vi "Vision Processing.vi"(4 "error in (no error)":errorcluster, 7 "Image Size":T1=enum."320x240") -> ()   [LabVIEW 2015]
doc: "This VI runs in parallel to other tasks. It gets images from the camera, processes them for color or shape and use that information to affect robot behavior."
uses:
  <vilib>/Rock Robotics/WPI/Camera/WPI_CameraImageSize.ctl
  <vilib>/vision/Image Controls.llb/IMAQ Image.ctl
  Program Files (x86)/National Instruments/LabVIEW 2015/examples/FRC/roboRIO/Vision/2016 Vision Example/Vision Support Code/Camera Types.ctl
  <vilib>/Rock Robotics/WPI/Camera/WPI_CameraWhite Balance Values.ctl
  <vilib>/Rock Robotics/WPI/Camera/WPI_CameraFrameRate.ctl
  <vilib>/Rock Robotics/WPI/Camera/WPI_CameraExposure Values.ctl
  Robot Global Data.vi
  Team Code/Global_Var/Drive_Global.vi
  <vilib>/vision/NI_Vision_Development_Module.lvlib
panel:
  out "Waveform Chart":dbl(graph)
  out "Vision_angle":cluster{"1":dbl, "2":dbl, "3":dbl}
  in  "Snap_Shot":bool
  in  "error in (no error) 2":errorcluster
  in  "Image Size 2":T1
  out "ms to process":u32=51
  in  "LED Color":T2={"Hue"={238.51289036032986, 17.562943497940463}, "Sat"={66.78571428571429, 255.0}, "Val"={48.571428571428584, 255.0}} {"Hue" scale=0.0..255.0 scale format="%#_3g"}
  out "Qualified Particles":i32
  in  "Score Threshold":dbl=75.0
  in  "Aspect Fudge Factor":dbl=1.0
  in  "Min Score Threshold":i32=75
  in  "Camera Type":T3=enum."MS HD3000 square"
  in  "Emphasize Limit Tests":bool=TRUE
  out "Masked 2":T4(plugin-control)
  in  "Display Mask":bool=TRUE
  out "Original Image":T4(plugin-control)
  in  "Display Original":bool=TRUE
  out "Sorted Particle Scores":T5(array[cluster]) {"Moment Factor" format="%#_3g"; "Aspect Ratio" format="%#_3g"; "Area to CH" format="%#_3g"; "X" format="%#_3g"; "Y" format="%#_3g"}
  out "Highest Avg Score":dbl
  out "Detected Targets":T6(array[cluster]) {"Normalized Rect"."Numeric 5" format="%#_2g"; "Normalized Rect"."Numeric 3" format="%#_2g"; "Normalized Rect"."Numeric 2" format="%#_2g"; "Normalized Rect"."Numeric" format="%#_2g"}
  out "fps":dbl=19.607843137254903
  out "Image Out":T4
  # "Density Profile"
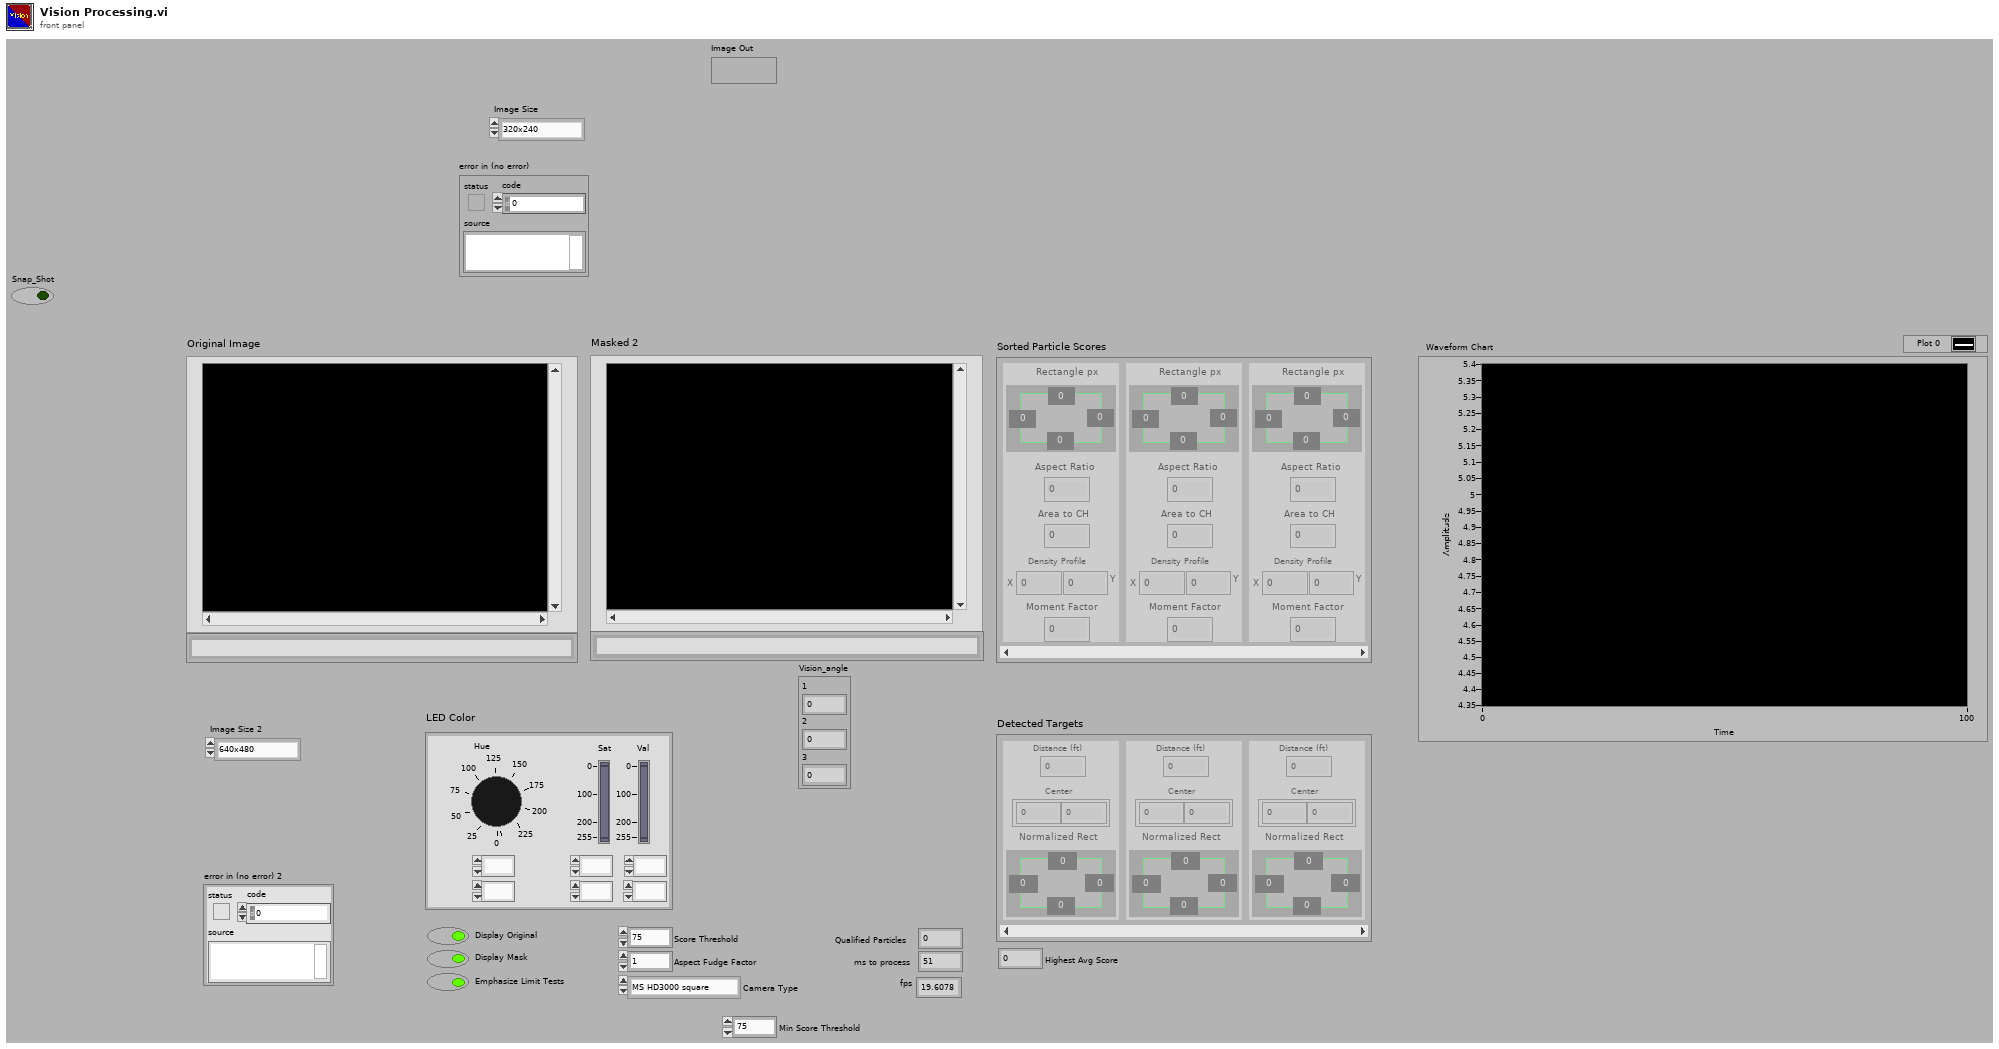
[diagram p1: front panel]
types:
  T1 = typedef "WPI_CameraImageSize.ctl" = enum16{"640x480", "320x240", "160x120", "Custom"}
  T2 = cluster{"Hue":cluster{dbl, dbl}, "Sat":cluster{dbl, dbl}, "Val":cluster{dbl, dbl}}
  T3 = typedef "Camera Types.ctl" = enum16{"206", "1011", "1013", "MS HD3000 square", "MS HD3000 640x480"}
  T4 = typedef "IMAQ Image.ctl" = refnum<image>
  T5 = cluster{"Rectangle px":cluster{"Numeric":dbl, "Numeric 2":dbl, "Numeric 3":dbl, "Numeric 5":dbl}, "Aspect Ratio":dbl, "Area to CH":dbl, "X":dbl, "Y":dbl, "Moment Factor":dbl}[]
  T6 = cluster{"Distance (ft)":dbl, "Center":cluster{dbl, dbl}, "Normalized Rect":cluster{"Numeric":dbl, "Numeric 2":dbl, "Numeric 3":dbl, "Numeric 5":dbl}}[]
  T7 = typedef "WPI_CameraExposure Values.ctl" = enum16{"Auto", "Flicker-free 50 Hz", "Flicker-free 60 Hz", "Hold current", "Custom"}
  T8 = typedef "WPI_CameraFrameRate.ctl" = u32
  T9 = typedef "WPI_CameraWhite Balance Values.ctl" = enum16{"Auto", "Fixed indoor", "Fixed outdoor 1", "Fixed outdoor 2", "Fixed fluorescent 1", "Fixed fluorescent 2", "Hold current", "Custom"}
  T10 = enum16{"Rising", "Falling", "Falling and Rising"}
  T11 = typedef "Particle Parameters" = i32
  T12 = typedef "Image Type" = u32
  T13 = typedef "WPI_CameraDevRef.ctl" = cluster{"Camera Address":string, "CameraStatus":errorcluster}
  T14 = cluster{"Bounding box":cluster{"left":dbl, "top":dbl, "right":dbl, "bottom":dbl}, "Aspect Ratio":dbl, "Area to CH":dbl, "X Mask":dbl, "Y Mask":dbl, "Moment":dbl}[]
  T15 = cluster{"Rectangle":cluster{"Numeric":dbl, "Numeric 2":dbl, "Numeric 3":dbl, "Numeric 5":dbl}, "L":dbl, "Area to CH":dbl, "X":dbl, "Y":dbl, "Moment Factor":dbl}[]
  T16 = cluster{"Distance (ft)":dbl, "Center":cluster{dbl, dbl}, "Normalized Rect":cluster{"Numeric":dbl, "Numeric 2":dbl, "Numeric 3":dbl, "Numeric 5":dbl}}
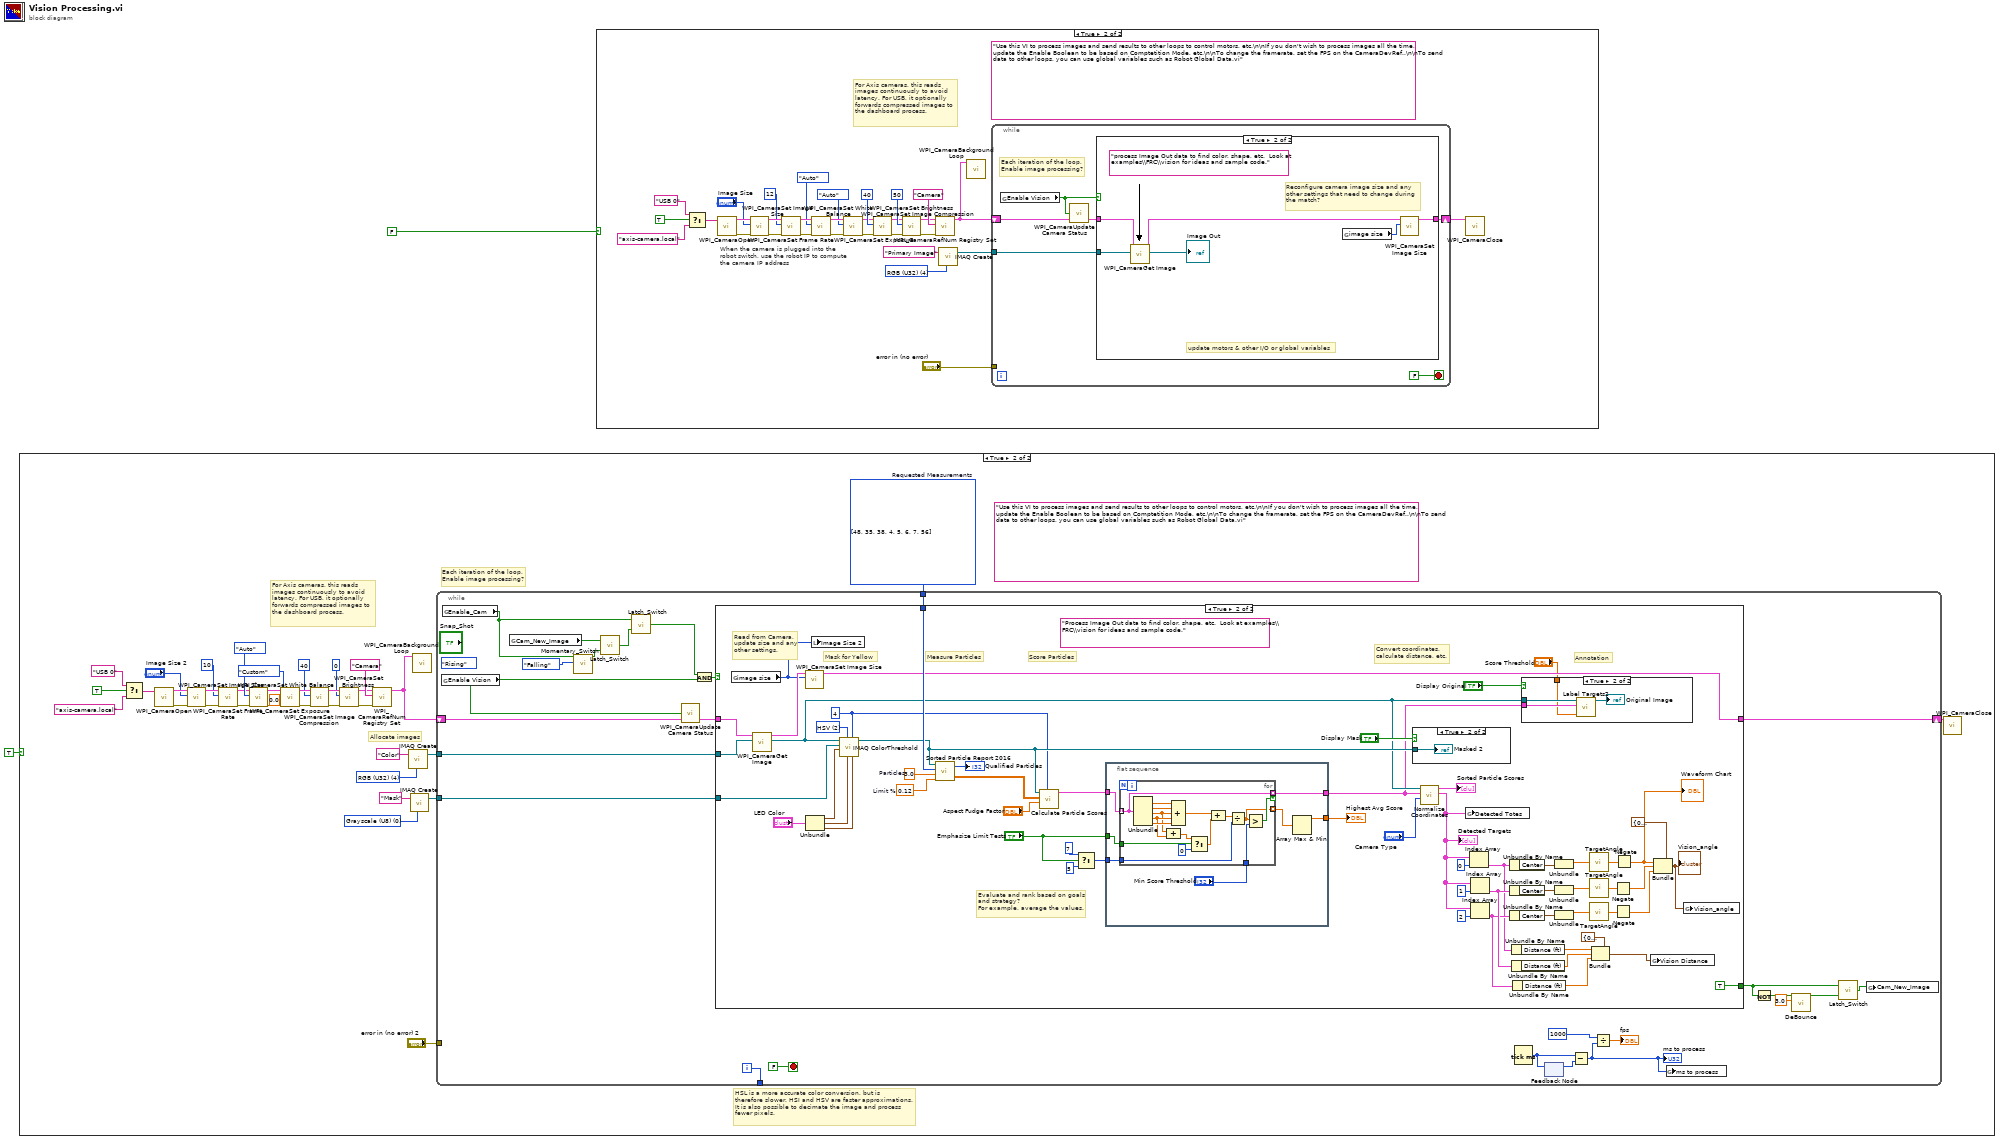
[diagram p0: block diagram]
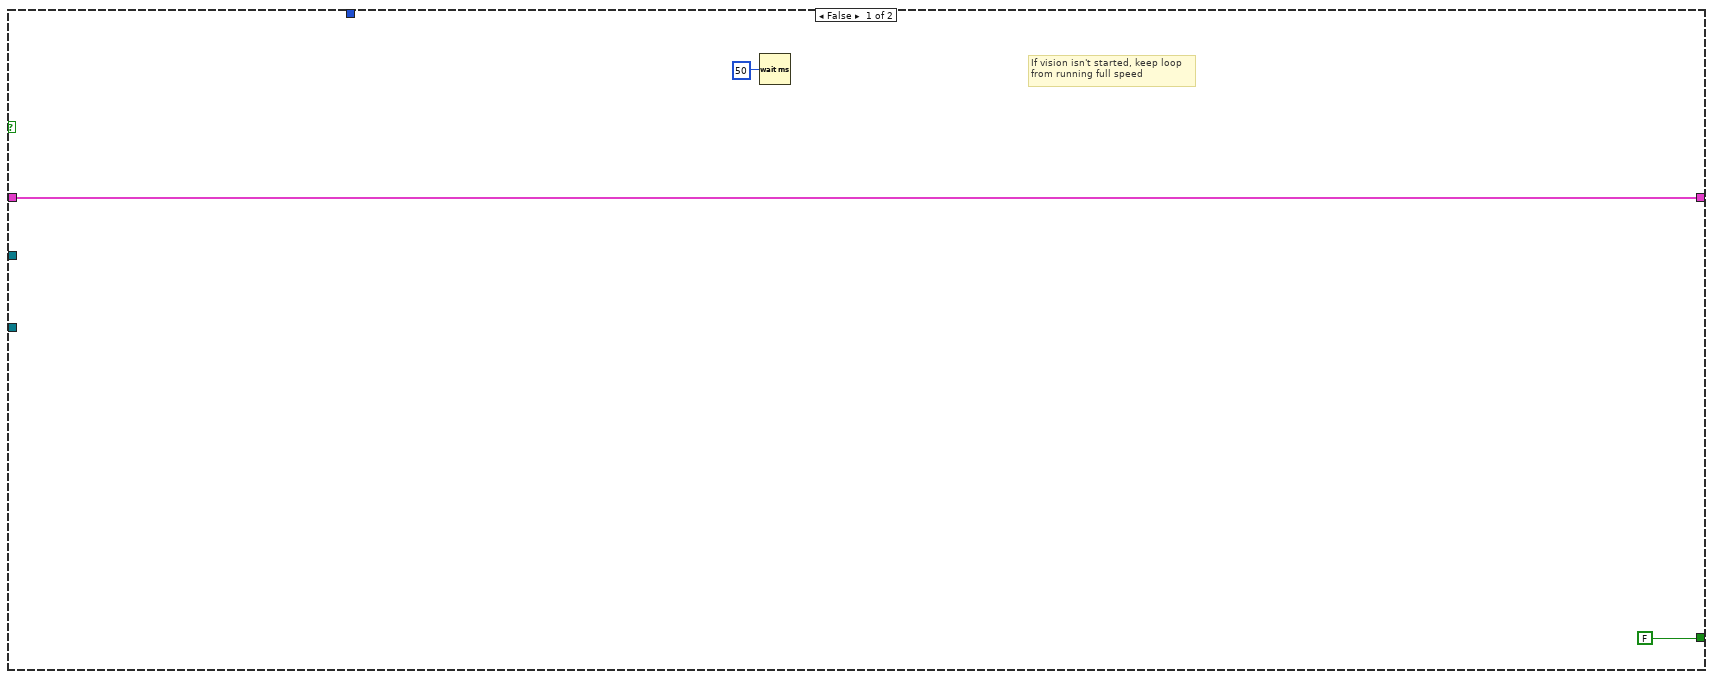
[diagram p3: hidden frame]
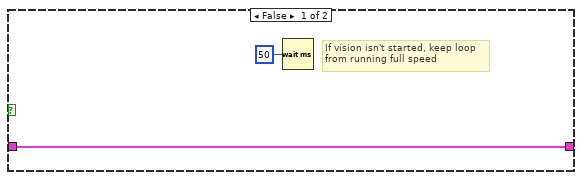
[diagram p7: hidden frame]
diagram:
  n1 = case shown="True" TRUE {
    frame False {
    }
    frame True {
      (unwired) "Use this VI to process images and send results to other loops to control motors, etc.\n\nIf you don't wish to process images all the time, update the Enable Boolean to be based on Comptetition Mode, etc.\n\nTo change the framerate, set the FPS on the CameraDevRef..\n\nTo send data to other loops, you can use global variables such as Robot Global Data.vi"
      w32 = T11[] [48, 35, 38, 4, 5, 6, 7, 56] items=["Center of Mass X", "Center of Mass Y", "First Pixel X", "First Pixel Y", "Bounding Rect Left", "Bounding Rect Top", "Bounding Rect Right", "Bounding Rect Bottom", "Max Feret Diameter Start X", "Max Feret Diameter Start Y", "Max Feret Diameter End X", "Max Feret Diameter End Y", "Max Horiz. Segment Length Left", "Max Horiz. Segment Length Right", "Max Horiz. Segment Length Row", "-", "Bounding Rect Width", "Bounding Rect Height", "Bounding Rect Diagonal", "Perimeter", "Convex Hull Perimeter", "Holes' Perimeter", "Max Feret Diameter", "Equivalent Ellipse Major Axis", "Equivalent Ellipse Minor Axis", "Equivalent Ellipse Minor Axis (Feret)", "Equivalent Rect Long Side", "Equivalent Rect Short Side", "Equivalent Rect Diagonal", "Equivalent Rect Short Side (Feret)", "Average Horiz. Segment Length", "Average Vert. Segment Length", "Hydraulic Radius", "Waddel Disk Diameter", "-", "Area", "Holes' Area", "Particle & Holes' Area", "Convex Hull Area", "Image Area", "-", "Number of Holes", "Number of Horiz. Segments", "Number of Vert. Segments", "-", "Orientation", "Max Feret Diameter Orientation", "-", "% Area/Image Area", "% Area/(Particle & Holes' Area)", "Ratio of Equivalent Ellipse Axes", "Ratio of Equivalent Rect Sides", "-", "Elongation Factor", "Compactness Factor", "Heywood Circularity Factor", "Type Factor", "-", "Sum X", "Sum Y", "Sum XX", "Sum XY", "Sum YY", "Sum XXX", "Sum XXY", "Sum XYY", "Sum YYY", "-", "Moment of Inertia XX", "Moment of Inertia XY", "Moment of Inertia YY", "Moment of Inertia XXX", "Moment of Inertia XXY", "Moment of Inertia XYY", "Moment of Inertia YYY", "Norm. Moment of Inertia XX", "Norm. Moment of Inertia XY", "Norm. Moment of Inertia YY", "Norm. Moment of Inertia XXX", "Norm. Moment of Inertia XXY", "Norm. Moment of Inertia XYY", "Norm. Moment of Inertia YYY", "Hu Moment 1", "Hu Moment 2", "Hu Moment 3", "Hu Moment 4", "Hu Moment 5", "Hu Moment 6", "Hu Moment 7"]  # Requested Measurements
      w35 = T12 0 items=["Grayscale (U8)", "Grayscale (I16)", "Grayscale (SGL)", "Complex (CSG)", "RGB (U32)", "HSL (U32)", "RGB (U64)", "Grayscale (U16)"] ("Image Type")
      w37 = T12 4 items=["Grayscale (U8)", "Grayscale (I16)", "Grayscale (SGL)", "Complex (CSG)", "RGB (U32)", "HSL (U32)", "RGB (U64)", "Grayscale (U16)"] ("Image Type")
      # "Each iteration of the loop,\nEnable image processing?"
      # "HSL is a more accurate color conversion, but is\ntherefore slower. HSI and HSV are faster approximations.\nIt is also possible to decimate the image and process\nfewer pixels."
      # "For Axis cameras, this reads\nimages continuously to avoid\nlatency. For USB, it optionally\nforwards compressed images to\nthe dashboard process."
      # "Allocate images"
      n2 = Select(t="USB 0" ("format string"), s=TRUE ("dot notation? (F)"), f="axis-camera.local" ("format string")) -> (s? t:f=w31:string)
      n3 = call <vilib>:"WPI_CameraOpen.vi"("Camera Address"=w31) -> ("error out"=w21:errorcluster, "CameraDevRef"=w20:T13)  [unwired: 1 in, 8 out]
      n4 = call <vilib>:"WPI_CameraSet Image Size.vi"("error in (no error)"=w21, "Image Size"="Image Size 2", "CameraDevRef"=w20) -> ("error out"=w22:errorcluster, "CameraDevRef Out"=w19:T13)  [unwired: 1 in, 6 out]
      n5 = call <vilib>:"WPI_CameraSet Frame Rate.vi"("error in (no error)"=w22, "Frame Rate (fps)"=T8 10, "CameraDevRef"=w19) -> ("error out"=w23:errorcluster, "CameraDevRef Out"=w17:T13)  [unwired: 7 out]
      n6 = call <vilib>:"WPI_CameraSet White Balance.vi"("error in (no error)"=w23, "White Balance"=WPI_CameraWhite_Balance_Values."Auto", "CameraDevRef"=w17) -> ("error out"=w24:errorcluster, "CameraDevRef Out"=w18:T13)  [unwired: 1 in, 6 out]
      n7 = call <vilib>:"WPI_CameraSet Exposure.vi"("error in (no error)"=w24, "Exposure (%)"=0.0, "Exposure"=WPI_CameraExposure_Values."Custom", "CameraDevRef"=w18) -> ("error out"=w25:errorcluster, "CameraDevRef Out"=w15:T13)  [unwired: 6 out]
      n8 = call <vilib>:"WPI_CameraSet Image Compression.vi"("error in (no error)"=w25, "Compression"=40, "CameraDevRef"=w15) -> ("error out"=w26:errorcluster, "CameraDevRef Out"=w16:T13)  [unwired: 7 out]
      n9 = call <vilib>:"WPI_CameraSet Brightness.vi"("error in (no error)"=w26, "Brightness"=0, "CameraDevRef"=w16) -> ("error out"=w27:errorcluster, "CameraDevRef Out"=w6:T13)  [unwired: 7 out]
      n10 = call <vilib>:"WPI_CameraRefNum Registry Set.vi"("error in (no error)"=w27, "refnum name"="Camera", "CameraDevRef"=w6) -> ("CameraDevRef"=w11:T13)  [unwired: 1 in, 7 out]
      n11 = call "IMAQ Create"("Image Name"="Color", "Image Type"=w37) -> ("New Image"=w36:T4)  [unwired: 2 in, 2 out]
      n12 = call "IMAQ Create"("Image Name"="Mask", "Image Type"=w35) -> ("New Image"=w33:T4)  [unwired: 2 in, 2 out]
      n13 = call <vilib>:"WPI_CameraBackground Loop.vi"("CameraDevRef"=w11) -> ()  [unwired: 11 in]
      n14 = while {
        tunnel: w36 -> [w59]
        tunnel: w33 -> [w63]
        tunnel: w32 -> [w62]
        tunnel: "error in (no error) 2" -> [_]
        tunnel: [w58] -> _
        shift-right: [w55] -> w7
        shift-left: w11 -> [w57]
        i -> [w58]
        stop <- FALSE stop-if-true
        (unwired) T10."Rising" ("Type")
        n15 = global read "Robot Global Data.vi" "Enable Vision"() -> (w51:bool)
        n16 = global read "Drive_Global.vi" "Enable_Cam"() -> (w47:bool)
        n17 = global read "Drive_Global.vi" "Cam_New_Image"() -> (w45:bool)
        n18 = call "Momentary_Switch.vi"("Type"=T10."Falling", "input_bol"=w47) -> ("out"=w50:bool)  [unwired: 9 in]
        n19 = call "Latch_Switch.vi"("Reset"=w50, "In"=w45) -> ("Out"=w48:bool)
        n20 = call "Latch_Switch.vi"("Reset"=w48, "In"=w47) -> ("Out"=w46:bool)
        n21 = call <vilib>:"WPI_CameraUpdate Camera Status.vi"("CameraDevRef In"=w57, "Enable Vision"=w51) -> ("CameraDevRef Out"=w56:T13)  [unwired: 3 in]
        n22 = And(x=w46, y=w51) -> (x .and. y?=w39:bool)
        n23 = case shown="True" w39 {
          tunnel: w63 -> [_ w126]
          tunnel: w62 -> [_ w121]
          tunnel: w56 -> [w66 w117]
          tunnel: w59 -> [_ w116]
          tunnel: [w66 w114] -> w55
          tunnel: [FALSE TRUE] -> w40
          frame False {
            # "If vision isn't started, keep loop\nfrom running full speed"
            n24 = Wait (ms)(milliseconds to wait=u32 50) -> ()  [unwired: 1 out]
          }
          frame True {
            w97 = 4 ("Replace Value")
            w111 = u16 2 items=["RGB", "HSL", "HSV", "HSI"] ("Color Mode")
            (unwired) "Process Image Out data to find color, shape, etc.  Look at examples\\FRC\\vision for ideas and sample code."
            w118 = 0.12  # Limit %
            w120 = 3.0  # Particles
            # "Evaluate and rank based on goals\nand strategy?\nFor example, average the values."
            # "Read from Camera,\nupdate size and any\nother settings."
            # "Measure Particles"
            # "Convert coordinates,\ncalculate distance, etc."
            # "Annotation"
            # "Score Particles"
            # "Mask for Yellow"
            n25 = global read "Robot Global Data.vi" "image size"() -> (w96:T1)
            n26 = call <vilib>:"WPI_CameraGet Image.vi"("Image"=w116, "CameraDevRef"=w117) -> ("Image Out"=w100:T4, "CameraDevRef Out"=w115:T13)  [unwired: 7 in, 1 out]
            n27 = call <vilib>:"WPI_CameraSet Image Size.vi"("Image Size"=w96, "CameraDevRef"=w115) -> ("CameraDevRef Out"=w114:T13)  [unwired: 2 in, 7 out]
            n28 = Unbundle("LED Color") -> ("Hue"=w125:cluster{dbl, dbl}, "Sat"=w124:cluster{dbl, dbl}, "Val"=w123:cluster{dbl, dbl})
            n29 = local write "Image Size 2"(w96) -> ()
            n30 = call "IMAQ ColorThreshold"("Blue or Luma or Val or Inten Range"=w123, "Replace Value"=w97, "Green or Sat Range"=w124, "Color Mode"=w111, "Red or Hue Range"=w125, "Image Dst"=w126, "Image Src"=w100) -> ("Image Dst Out"=w110:T4)  [unwired: 3 in, 1 out]
            n31 = call "Sorted Particle Report 2016.vi"("Min Area Size %"=w118, "Particle Count Limit"=w120, "Pixel Measurements"=w121, "Image in"=w110) -> ("Sorted Data"=w109:dbl[][], "Particles"=→"Qualified Particles":i32)
            n32 = call "Calculate Particle Scores.vi"("Pixel Value"=w97, "Aspect Fudge Factor"="Aspect Fudge Factor", "Sorted Data"=w109, "Image in"=w110) -> ("Scores"=w107:T14)  [unwired: 7 in]
            n33 = Select(t=7, s="Emphasize Limit Tests", f=5) -> (s? t:f=w104:i32)
            n34 = flat-sequence {
              tunnel: w107 -> [w137]
              tunnel: w104 -> [w135]
              tunnel: [w138] -> w103
              tunnel: [w132] -> w99
              tunnel: "Emphasize Limit Tests" -> [w136]
              frame #0 {
                n35 = for {
                  tunnel: w137 -> [w152] mode=indexing
                  tunnel: [w152] -> w132 mode=indexing if=w151
                  tunnel: [w150] -> w133 mode=indexing
                  tunnel: w135 -> [w149]
                  tunnel: "Min Score Threshold" -> [w148]
                  tunnel: w136 -> [w141]
                  n36 = Unbundle(w152) -> ("Aspect Ratio"=w154:dbl, "Area to CH"=w153:dbl, "X Mask"=w143:dbl, "Y Mask"=w144:dbl, "Moment"=w145:dbl)  [unwired: 1 out]
                  n37 = Compound Arithmetic op=ADD(w143, w144) -> (w142:dbl)
                  n38 = Compound Arithmetic op=ADD(w154, w153, w143, w144, w145) -> (w147:dbl)
                  n39 = Select(t=w142, s=w141, f=0) -> (s? t:f=w140:dbl)
                  n40 = Compound Arithmetic op=ADD(w147, w140) -> (w146:dbl)
                  n41 = Divide(x=w146, y=w149) -> (x/y=w150:dbl)
                  n42 = Greater?(x=w150, y=w148) -> (0:w151:bool)
                }
                n43 = Array Max & Min(array=w133) -> (max value=w138:dbl)  [unwired: 3 out]
              }
            }
            n44 = case shown="True" "Display Mask" {
              tunnel: w110 -> [_ w131]
              frame False {
              }
              frame True {
                "Masked 2" <- w131
              }
            }
            n45 = call "Normalize Coordinates.vi"("Camera Type"="Camera Type", "Targets"=w99, "Image in"=w100) -> ("Found Targets"=w91:T6, "Sorted Scores"=→"Sorted Particle Scores":T15)  [unwired: 7 in]
            "Detected Targets" <- w91
            n46 = global write "Robot Global Data.vi" "Detected Totes"(w91) -> ()
            n47 = Index Array(array=w91, index=0) -> (element=w68:T16)
            n48 = Index Array(array=w91, index=1) -> (element=w82:T16)
            n49 = Index Array(array=w91, index=2) -> (element=w81:T16)
            n50 = Unbundle By Name(w68) -> ("Center"=w90:cluster{dbl, dbl})
            n51 = Unbundle By Name(w82) -> ("Center"=w89:cluster{dbl, dbl})
            n52 = Unbundle By Name(w81) -> ("Center"=w88:cluster{dbl, dbl})
            n53 = Unbundle By Name(w68) -> ("Distance (ft)"=w80:dbl)
            n54 = Unbundle By Name(w82) -> ("Distance (ft)"=w79:dbl)
            n55 = Unbundle By Name(w81) -> ("Distance (ft)"=w78:dbl)
            n56 = case shown="True" "Display Original" {
              tunnel: w100 -> [_ w130]
              tunnel: w99 -> [_ w128]
              tunnel: "Score Threshold" -> [_ w127]
              frame False {
              }
              frame True {
                n57 = call "Label Targets2.vi"("Score Threshold"=w127, "Targets"=w128, "Image in"=w130) -> ("Image out"=→"Original Image":T4)  [unwired: 8 in]
              }
            }
            n58 = Unbundle(w90) -> (w87:dbl)  [unwired: 1 out]
            n59 = Unbundle(w89) -> (w86:dbl)  [unwired: 1 out]
            n60 = Unbundle(w88) -> (w85:dbl)  [unwired: 1 out]
            n61 = call "TargetAngle.vi"("Horizontal_Pixel"=w87) -> ("TargetAngle"=w75:dbl)
            n62 = call "TargetAngle.vi"("Horizontal_Pixel"=w86) -> ("TargetAngle"=w74:dbl)
            n63 = call "TargetAngle.vi"("Horizontal_Pixel"=w85) -> ("TargetAngle"=w72:dbl)
            n64 = Bundle(cluster=cluster{"1":dbl, "2":dbl, "3":dbl} {"1"=0.0, "2"=0.0, "3"=0.0}, "1"=w80, "2"=w79, "3"=w78) -> (w76:cluster{"1":dbl, "2":dbl, "3":dbl})
            n65 = Negate(x=w74) -> (-x=w73:dbl)
            n66 = Negate(x=w72) -> (-x=w71:dbl)
            n67 = Negate(x=w75) -> (-x=w70:dbl)
            "Waveform Chart" <- w70
            n68 = global write "Drive_Global.vi" "Vision Distance"(w76) -> ()
            n69 = Bundle(cluster=cluster{"1":dbl, "2":dbl, "3":dbl} {"1"=0.0, "2"=0.0, "3"=0.0}, "1"=w70, "2"=w73, "3"=w71) -> (w83:cluster{"1":dbl, "2":dbl, "3":dbl})
            "Vision_angle" <- w83
            n70 = global write "Drive_Global.vi" "Vision_angle"(w83) -> ()
            "Highest Avg Score" <- w103
          }
        }
        n71 = Tick Count (ms)() -> (millisecond timer value=w60:u32)
        n72 = feedback-in #1(w60) -> ()
        n73 = feedback #1() -> (w61:u32)  [unwired: 1 in]
        n74 = Subtract(x=w60, y=w61) -> (x-y=w54:u32)
        "ms to process" <- w54
        n75 = Divide(x=1000 ("Brightness"), y=w54) -> (x/y=→"fps":dbl)
        n76 = global write "Robot Global Data.vi" "ms to process"(w54) -> ()
        n77 = Not(x=w40) -> (.not. x?=w43:bool)
        n78 = call "DeBounce.vi"("DB_Count"=3.0, "Value"=w43) -> ("BD_Value"=w44:bool)  [unwired: 9 in]
        n79 = call "Latch_Switch.vi"("Reset"=w44, "In"=w40) -> ("Out"=w41:bool)
        n80 = global write "Drive_Global.vi" "Cam_New_Image"(w41) -> ()
      }
      n81 = call <vilib>:"WPI_CameraClose.vi"("CameraDevRef"=w7) -> ()  [unwired: 1 in, 10 out]
    }
  }
  n82 = case shown="True" FALSE {
    frame False {
    }
    frame True {
      (unwired) "Use this VI to process images and send results to other loops to control motors, etc.\n\nIf you don't wish to process images all the time, update the Enable Boolean to be based on Comptetition Mode, etc.\n\nTo change the framerate, set the FPS on the CameraDevRef..\n\nTo send data to other loops, you can use global variables such as Robot Global Data.vi"
      w185 = T12 4 items=["Grayscale (U8)", "Grayscale (I16)", "Grayscale (SGL)", "Complex (CSG)", "RGB (U32)", "HSL (U32)", "RGB (U64)"] ("Image Type")
      # "When the camera is plugged into the\nrobot switch, use the robot IP to compute\nthe camera IP address"
      # "For Axis cameras, this reads\nimages continuously to avoid\nlatency. For USB, it optionally\nforwards compressed images to\nthe dashboard process."
      n83 = Select(t="USB 0" ("format string"), s=TRUE ("dot notation? (F)"), f="axis-camera.local" ("format string")) -> (s? t:f=w156:string)
      n84 = call <vilib>:"WPI_CameraOpen.vi"("Camera Address"=w156) -> ("error out"=w173:errorcluster, "CameraDevRef"=w174:T13)  [unwired: 1 in, 8 out]
      n85 = call <vilib>:"WPI_CameraSet Image Size.vi"("error in (no error)"=w173, "Image Size"="Image Size", "CameraDevRef"=w174) -> ("error out"=w172:errorcluster, "CameraDevRef Out"=w175:T13)  [unwired: 1 in, 6 out]
      n86 = call <vilib>:"WPI_CameraSet Frame Rate.vi"("error in (no error)"=w172, "Frame Rate (fps)"=T8 12, "CameraDevRef"=w175) -> ("error out"=w171:errorcluster, "CameraDevRef Out"=w177:T13)  [unwired: 7 out]
      n87 = call <vilib>:"WPI_CameraSet White Balance.vi"("error in (no error)"=w171, "White Balance"=WPI_CameraWhite_Balance_Values."Auto", "CameraDevRef"=w177) -> ("error out"=w170:errorcluster, "CameraDevRef Out"=w176:T13)  [unwired: 1 in, 6 out]
      n88 = call <vilib>:"WPI_CameraSet Exposure.vi"("error in (no error)"=w170, "Exposure"=WPI_CameraExposure_Values."Auto", "CameraDevRef"=w176) -> ("error out"=w169:errorcluster, "CameraDevRef Out"=w179:T13)  [unwired: 1 in, 6 out]
      n89 = call <vilib>:"WPI_CameraSet Image Compression.vi"("error in (no error)"=w169, "Compression"=40, "CameraDevRef"=w179) -> ("error out"=w168:errorcluster, "CameraDevRef Out"=w178:T13)  [unwired: 7 out]
      n90 = call <vilib>:"WPI_CameraSet Brightness.vi"("error in (no error)"=w168, "Brightness"=50, "CameraDevRef"=w178) -> ("error out"=w166:errorcluster, "CameraDevRef Out"=w167:T13)  [unwired: 7 out]
      n91 = call <vilib>:"WPI_CameraRefNum Registry Set.vi"("error in (no error)"=w166, "refnum name"="Camera", "CameraDevRef"=w167) -> ("CameraDevRef"=w162:T13)  [unwired: 1 in, 7 out]
      n92 = call "IMAQ Create"("Image Name"="Primary Image", "Image Type"=w185) -> ("New Image"=w183:T4)  [unwired: 2 in, 2 out]
      n93 = call <vilib>:"WPI_CameraBackground Loop.vi"("CameraDevRef"=w162) -> ()  [unwired: 11 in]
      n94 = while {
        shift-right: [w190] -> w160
        shift-left: w162 -> [w188]
        tunnel: w183 -> [w189]
        tunnel: "error in (no error)" -> [_]
        stop <- FALSE stop-if-true
        # "Each iteration of the loop,\nEnable image processing?"
        n95 = global read "Robot Global Data.vi" "Enable Vision"() -> (w186:bool)
        n96 = call <vilib>:"WPI_CameraUpdate Camera Status.vi"("CameraDevRef In"=w188, "Enable Vision"=w186) -> ("CameraDevRef Out"=w187:T13)  [unwired: 3 in]
        n97 = case shown="True" w186 {
          tunnel: w189 -> [_ w198]
          tunnel: [w193 w199] -> w190
          tunnel: w187 -> [w193 w196]
          frame False {
            # "If vision isn't started, keep loop\nfrom running full speed"
            n98 = Wait (ms)(milliseconds to wait=u32 50) -> ()  [unwired: 1 out]
          }
          frame True {
            (unwired) "process Image Out data to find color, shape, etc.  Look at examples\\FRC\\vision for ideas and sample code."
            # "update motors & other I/O or global variables"
            # "Reconfigure camera image size and any\nother settings that need to change during\nthe match?"
            n99 = call <vilib>:"WPI_CameraGet Image.vi"("Image"=w198, "CameraDevRef"=w196) -> ("Image Out"=→"Image Out":T4, "CameraDevRef Out"=w195:T13)  [unwired: 1 in, 7 out]
            n100 = global read "Robot Global Data.vi" "image size"() -> (w197:T1)
            n101 = call <vilib>:"WPI_CameraSet Image Size.vi"("Image Size"=w197, "CameraDevRef"=w195) -> ("CameraDevRef Out"=w199:T13)  [unwired: 2 in, 7 out]
          }
        }
      }
      n102 = call <vilib>:"WPI_CameraClose.vi"("CameraDevRef"=w160) -> ()  [unwired: 1 in, 10 out]
    }
  }
